vi "ClassifyBlobs.vi"(10 "Horizontal Targets":T2[](array[typedef]) {"Particle Report"."Equiv. Rect"."Height" format="%.2f"; "Particle Report"."Equiv. Rect"."Width" format="%.2f"; "Particle Report"."Center of Mass"."Y" format="%.2f"; "Particle Report"."Center of Mass"."X" format="%.2f"; "Particle Report"."Bounding Rect"."Bottom" format="%.2f"; "Particle Report"."Bounding Rect"."Right" format="%.2f"; "Particle Report"."Bounding Rect"."Top" format="%.2f"; "Particle Report"."Bounding Rect"."Left" format="%.2f"; "Particle Report"."Area" format="%.2f"}, 11 "Vertical Target":T2 {"Particle Report"."Equiv. Rect"."Height" format="%.2f"; "Particle Report"."Equiv. Rect"."Width" format="%.2f"; "Particle Report"."Center of Mass"."Y" format="%.2f"; "Particle Report"."Center of Mass"."X" format="%.2f"; "Particle Report"."Bounding Rect"."Bottom" format="%.2f"; "Particle Report"."Bounding Rect"."Right" format="%.2f"; "Particle Report"."Bounding Rect"."Top" format="%.2f"; "Particle Report"."Bounding Rect"."Left" format="%.2f"; "Particle Report"."Area" format="%.2f"}) -> (3 "Scores":T1[](array[typedef]))   [LabVIEW 2013]
uses:
  ScoredBlobType.ctl
  BlobMeasurementType.ctl
  CombinedScore.ctl
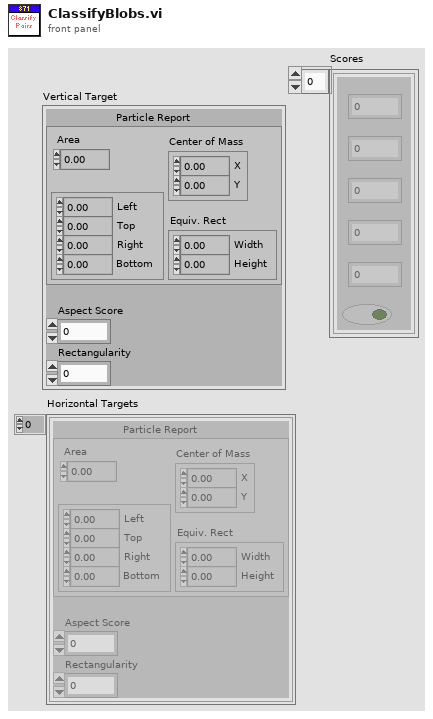
[diagram p1: front panel]
types:
  T1 = typedef "CombinedScore.ctl" = cluster{"Left Score":dbl, "Right Score":dbl, "Ratio Score":dbl, "Vert Score":dbl, "Index":i32, "Hot?":bool}
  T2 = typedef "ScoredBlobType.ctl" = cluster{"Particle Report":T3, "Aspect Score":dbl, "Rectangularity":dbl}
  T3 = typedef "BlobMeasurementType.ctl" = cluster{"Area":dbl, "Bounding Rect":cluster{"Left":dbl, "Top":dbl, "Right":dbl, "Bottom":dbl}, "Center of Mass":cluster{"X":dbl, "Y":dbl}, "Equiv. Rect":cluster{"Width":dbl, "Height":dbl}}
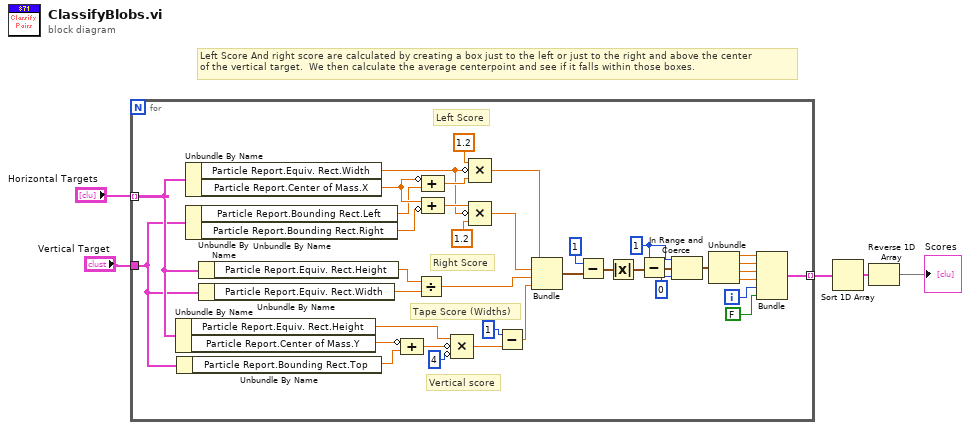
[diagram p0: block diagram]
diagram:
  # "Left Score And right score are calculated by creating a box just to the left or just to the right and above the center \nof the vertical target.  We then calculate the average centerpoint and see if it falls within those boxes."
  n1 = for {
    tunnel: "Horizontal Targets" -> [w10] mode=indexing
    tunnel: "Vertical Target" -> [w8]
    tunnel: [w25] -> w5 mode=indexing
    i -> [w20]
    w29 = 1
    # "Vertical score"
    # "Tape Score (Widths)"
    # "Right Score"
    # "Left Score"
    n2 = Unbundle By Name(w10) -> ("Particle Report.Equiv. Rect.Height"=w11:dbl, "Particle Report.Center of Mass.Y"=w13:dbl)
    n3 = Unbundle By Name(w8) -> ("Particle Report.Bounding Rect.Top"=w14:dbl)
    n4 = Unbundle By Name(w10) -> ("Particle Report.Equiv. Rect.Width"=w39:dbl, "Particle Report.Center of Mass.X"=w15:dbl)
    n5 = Unbundle By Name(w8) -> ("Particle Report.Bounding Rect.Left"=w7:dbl, "Particle Report.Bounding Rect.Right"=w6:dbl)
    n6 = Unbundle By Name(w10) -> ("Particle Report.Equiv. Rect.Height"=w9:dbl)
    n7 = Unbundle By Name(w8) -> ("Particle Report.Equiv. Rect.Width"=w38:dbl)
    n8 = Compound Arithmetic op=ADD(invert w13, w14) -> (w12:dbl)
    n9 = Divide(x=w9, y=w38) -> (x/y=w35:dbl)
    n10 = Compound Arithmetic op=ADD(invert w15, w7) -> (w42:dbl)
    n11 = Compound Arithmetic op=ADD(w15, invert w6) -> (w41:dbl)
    n12 = Compound Arithmetic op=MULTIPLY(w11, invert w12, invert 4) -> (w18:dbl)
    n13 = Compound Arithmetic op=MULTIPLY(1.2, invert w39, w42) -> (w36:dbl)
    n14 = Compound Arithmetic op=MULTIPLY(w41, invert w39, 1.2) -> (w34:dbl)
    n15 = Subtract(x=1, y=w18) -> (x-y=w17:dbl)
    n16 = Bundle(w36, w34, w35, w17) -> (w33:cluster{dbl, dbl, dbl, dbl})  [unwired: 1 in]
    n17 = Subtract(x=1, y=w33) -> (x-y=w31:cluster{dbl, dbl, dbl, dbl})
    n18 = Absolute Value(x=w31) -> (abs(x)=w30:cluster{dbl, dbl, dbl, dbl})
    n19 = Subtract(x=w29, y=w30) -> (x-y=w28:cluster{dbl, dbl, dbl, dbl})
    n20 = In Range and Coerce(upper limit=w29, x=w28, lower limit=0) -> (coerced(x)=w26:cluster{dbl, dbl, dbl, dbl})  [unwired: 1 out]
    n21 = Unbundle(w26) -> (w24:dbl, w23:dbl, w22:dbl, w21:dbl)
    n22 = Bundle(w24, w23, w22, w21, w20, FALSE) -> (w25:cluster{dbl, dbl, dbl, dbl, i32, bool})  [unwired: 1 in]
  }
  n23 = Sort 1D Array(array=w5) -> (sorted array=w4:cluster{dbl, dbl, dbl, dbl, i32, bool}[])
  n24 = Reverse 1D Array(array=w4) -> (reversed array=→"Scores":cluster{dbl, dbl, dbl, dbl, i32, bool}[])
